vi "Get Valid Channel Value String.vi"(10 "Digital":bool=TRUE, 11 "Channel Values":string) -> (3 "Valid Channel Values":string)   [LabVIEW 2024]
uses:
  Global Strings.vi
  Sequencer with Output Values.lvclass
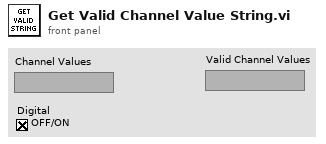
[diagram p1: front panel]
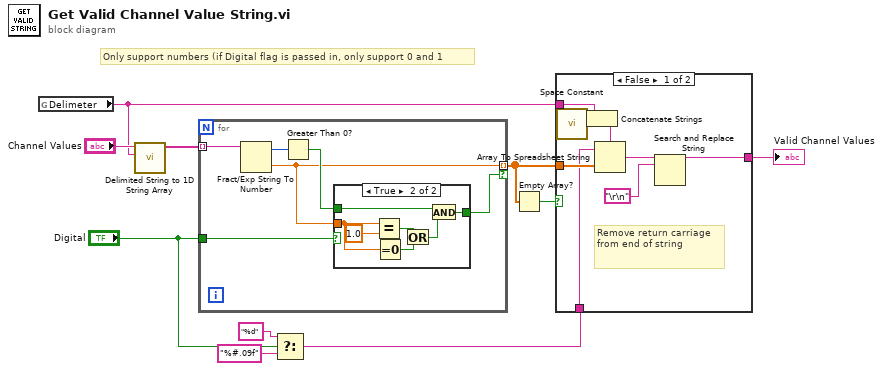
[diagram p0: block diagram]
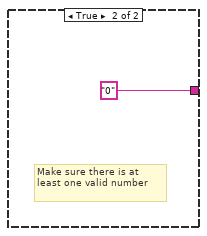
[diagram p2: hidden frame]
diagram:
  # "Only support numbers (if Digital flag is passed in, only support 0 and 1"
  n1 = global read "Global Strings.vi" "Delimeter"() -> (w1:string)
  n2 = call <vilib>:"Delimited String to 1D String Array.vi"("delimiter"=w1, "delimited string"="Channel Values") -> ("string array"=w9:string[])  [unwired: 9 in]
  n3 = for {
    tunnel: w9 -> [w16] mode=indexing
    tunnel: "Digital" -> [w14]
    tunnel: [w12] -> w7 mode=indexing if=w11
    n4 = Fract/Exp String To Number(string=w16) -> (offset past number=w15:i32, number=w12:dbl)  [unwired: 3 in]
    n5 = Greater Than 0?(x=w15) -> (x > 0?=w13:bool)
    n6 = case shown="True" w14 {
      tunnel: w13 -> [w17 w20]
      tunnel: w12 -> [_ w23]
      tunnel: [w17 w18] -> w11
      frame False {
      }
      frame True {
        n7 = Equal?(x=w23, y=1.0) -> (x = y?=w22:bool)
        n8 = Equal To 0?(x=w23) -> (x = 0?=w21:bool)
        n9 = Or(x=w22, y=w21) -> (x .or. y?=w19:bool)
        n10 = And(x=w20, y=w19) -> (x .and. y?=w18:bool)
      }
    }
  }
  n11 = Select(t="%d", s="Digital", f="%#.09f") -> (s? t:f=w3:string)
  n12 = Empty Array?(array=w7) -> (empty?=w8:bool)
  n13 = case shown="False" w8 {
    tunnel: w7 -> [w32 _]
    tunnel: w3 -> [w31 _]
    tunnel: w1 -> [w27 _]
    tunnel: [w28 "0" ("result string")] -> w2
    frame False {
      # "Remove return carriage from end of string"
      n14 = call <vilib>:"Space Constant.vi"() -> ("String"=w26:string)
      n15 = Concatenate Strings(w27, w26) -> (w25:string)
      n16 = Array To Spreadsheet String(delimiter (Tab)=w25, array=w32, 3:w31) -> (spreadsheet string=w30:string)
      n17 = Search and Replace String(input string=w30, search string="\r\n") -> (result string=w28:string)  [unwired: 6 in, 3 out]
    }
    frame True {
      # "Make sure there is at least one valid number"
    }
  }
  "Valid Channel Values" <- w2
